vi "Get SMO Port.vi"(8 "error in (no error)":errorcluster, 11 "ExampleInstrument in":refnum<class "LevyLab Instrument.lvclass">) -> (0 "error out":errorcluster, 2 "Port":u16, 3 "ExampleInstrument out":refnum<class "LevyLab Instrument.lvclass">)   [LabVIEW 2016, in "LevyLab Instrument.lvclass"]
uses:
  LevyLab Instrument.lvclass
  SMOs/Instrument/Instrument.lvclass
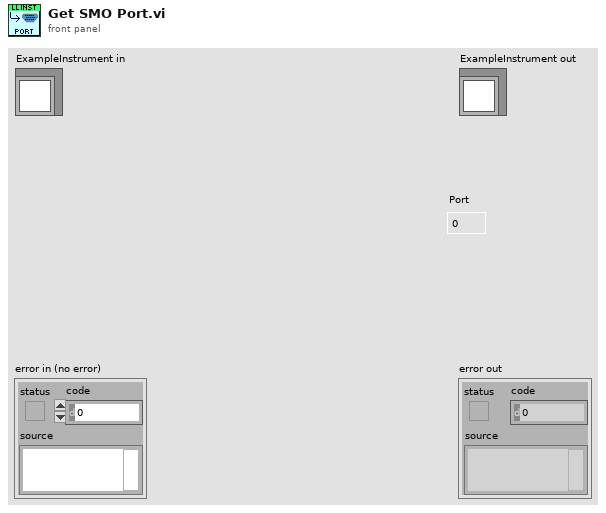
[diagram p1: front panel]
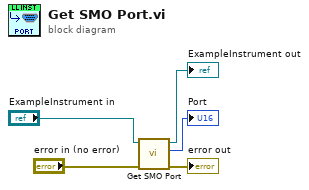
[diagram p0: block diagram]
diagram:
  n1 = call-parent "Get SMO Port.vi"("error in (no error)"="error in (no error)", "Instrument in"="ExampleInstrument in") -> ("error out"=→"error out":errorcluster, "Port"=→"Port":u16, "Instrument out"=→"ExampleInstrument out":refnum<class "LevyLab Instrument.lvclass">)  [unwired: 7 in]
